vi "Init Hardware.vi"(8 "error in (no error)":errorcluster, 11 "Ocean Optics Driver in":refnum<class "Ocean Optics Driver.lvclass">) -> (0 "error out":errorcluster, 3 "Ocean Optics Driver out":refnum<class "Ocean Optics Driver.lvclass">)   [LabVIEW 2016, in "Ocean Optics Driver.lvclass"]
uses:
  Ocean Optics Driver.lvclass
  C:/github/NHMFL_Core/Libraries/Instruments/VISA Instrument/VISA Instrument.lvclass
  C:/github/NHMFL_Core/Libraries/Instruments/Spectrometer Driver/Spectrometer Driver.lvclass
  VISA Instrument/VISA Instrument.lvclass/VISA Instrument.ctl
  Spectrometer Driver/Spectrometer Driver.lvclass/Spectrometer Driver.ctl
  VISA Instrument/Read VISA resource.vi
  VISA Instrument/Write VISA resource.vi
  Spectrometer Driver/Write Wavelengths.vi
  Read Ocean optics configuration.vi
  <instrlib>/Ocean Optics 2000 4000/Ocean Optics 2000 4000.lvlib
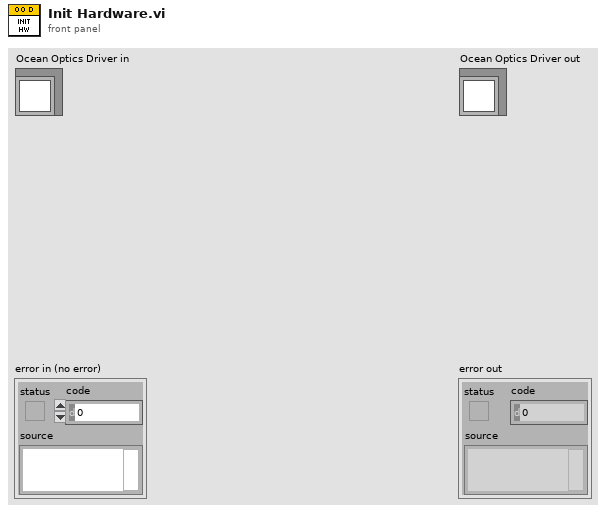
[diagram p1: front panel]
types:
  T1 = typedef "Ocean optics configuration.ctl" = cluster{"Integration time":dbl, "Fit parameters":T2, "Fit":bool, "Use last fit as  guess":bool, "Window width":dbl, "Repeat":i32, "Reference wavelengh":dbl}
  T2 = typedef "Multi-peak Parameters.ctl" = cluster{"Peaks":T3[], "Slope":dbl, "Intercept":dbl, "Function":enum16{"Gauss", "Lorentz"}}
  T3 = typedef "Peak Parameters.ctl" = cluster{"Amplitude":dbl, "Center":dbl, "Width":dbl}
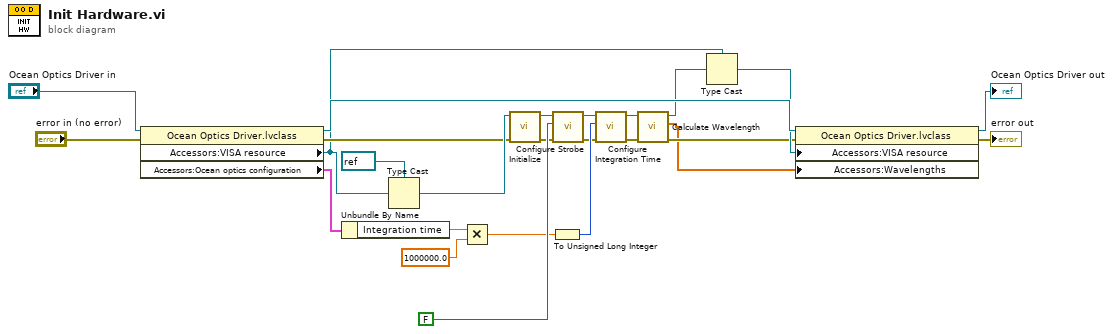
[diagram p0: block diagram]
diagram:
  n1 = property class="Ocean Optics Driver.lvclass"(reference="Ocean Optics Driver in", error in="error in (no error)") -> (reference out=w8:refnum<class "Ocean Optics Driver.lvclass">, error out=w21:errorcluster, "Accessors:VISA resource"=w6:refnum<visa-resource-name>, "Accessors:Ocean optics configuration"=w24:T1)
  n2 = Unbundle By Name(w24) -> ("Integration time"=w10:dbl)
  n3 = Type Cast(type=refnum<visa-resource-name> refnum ("VISA resource name"), x=w6) -> (*(type *) &x=w22:refnum<visa-resource-name>)
  n4 = Multiply(x=w10, y=1000000.0) -> (x*y=w18:dbl)
  n5 = call <instrlib>:"Initialize.vi"("error in (no error)"=w21, "VISA resource name"=w22) -> ("error out"=w11:errorcluster, "VISA resource name out"=w12:refnum<visa-resource-name>)  [unwired: 1 in, 7 out]
  n6 = To Unsigned Long Integer(number=w18) -> (unsigned 32bit integer=w19:u32)
  n7 = call <instrlib>:"Configure Strobe.vi"("error in (no error)"=w11, "Enable Strobe (Disabled)"=FALSE, "VISA resource name"=w12) -> ("error out"=w14:errorcluster, "VISA resource name out"=w13:refnum<visa-resource-name>)  [unwired: 7 out]
  n8 = call <instrlib>:"Configure Integration Time.vi"("error in (no error)"=w14, "Integration Time (6000)"=w19, "VISA resource name"=w13) -> ("error out"=w15:errorcluster, "VISA resource name out"=w16:refnum<visa-resource-name>)  [unwired: 7 in]
  n9 = call <instrlib>:"Calculate Wavelength.vi"("error in (no error)"=w15, "VISA resource name"=w16) -> ("error out"=w4:errorcluster, "Wavelength (nm)"=w1:dbl[], "VISA resource name out"=w7:refnum<visa-resource-name>)  [unwired: 1 in, 6 out]
  n10 = Type Cast(type=w6, x=w7) -> (*(type *) &x=w5:refnum<visa-resource-name>)
  n11 = property class="Ocean Optics Driver.lvclass"(reference=w8, error in=w4, "Accessors:VISA resource"=w5, "Accessors:Wavelengths"=w1) -> (reference out=→"Ocean Optics Driver out":refnum<class "Ocean Optics Driver.lvclass">, error out=→"error out":errorcluster)
